vi "GetCoordinates.vi"(8 "error in (no error)":errorcluster, 11 "Snake in":refnum<class "Snake.lvclass">) -> (0 "error out":errorcluster, 2 "Coordinates":T1[](array[typedef]), 3 "Snake out":refnum<class "Snake.lvclass">)   [LabVIEW 2019, in "RT_Game.lvlib" / "Snake.lvclass"]
uses:
  Snake.lvclass
  Game/Coordinate.ctl
  Snake.lvclass/Snake.ctl
  Game/Game.lvclass
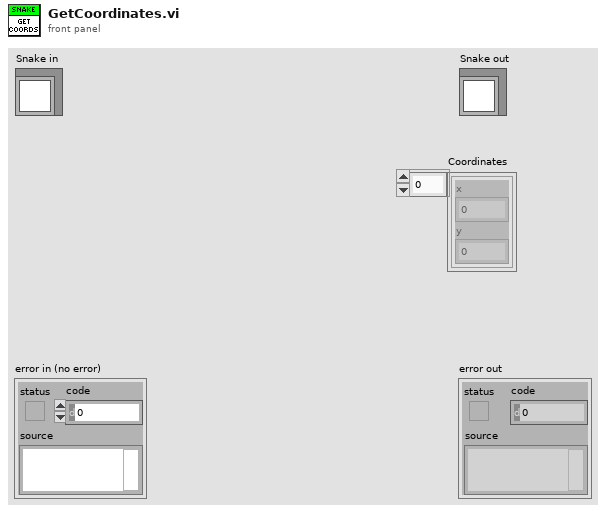
[diagram p1: front panel]
types:
  T1 = typedef "RT_Game.lvlib/Game.lvclass/Coordinate.ctl" = cluster{"x":dbl, "y":dbl}
  T2 = typedef "RT_Game.lvlib/SnakeGame.lvclass/CoordinateData.ctl" = cluster{"Coordinate":T1, "TileCode":u16}
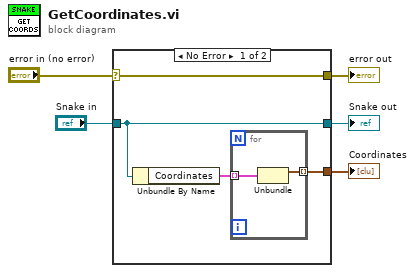
[diagram p0: block diagram]
diagram:
  n1 = case shown="No Error" "error in (no error)" {
    selector: "error in (no error)" -> [w9 w13]
    tunnel: [w9 w13] -> w4
    tunnel: [w8 w12] -> w2
    tunnel: "Snake in" -> [w8 w12]
    tunnel: [w6 _] -> w1
    frame No Error {
      n2 = Unbundle By Name(w8) -> ("Coordinates"=w7:T2[])
      n3 = for {
        tunnel: w7 -> [w11] mode=indexing
        tunnel: [w10] -> w6 mode=indexing
        n4 = Unbundle(w11) -> ("Coordinate"=w10:T1)  [unwired: 1 out]
      }
    }
    frame Error {
    }
  }
  "error out" <- w4
  "Snake out" <- w2
  "Coordinates" <- w1
